vi "lfieldpanel_store_sequence.vi"(6 "dset_name":string, 7 "image_data":T1, 8 "error in (no error)":errorcluster, 9 "notes":string, 10 "Path":path, 11 "lightfield_panel in":refnum<class "lightfield_panel.lvclass">) -> (0 "error out":errorcluster, 3 "lightfield_panel out":refnum<class "lightfield_panel.lvclass">)   [LabVIEW 2015, in "lightfield_panel.lvclass"]
uses:
  lightfield_panel.lvclass
  lightfield_panel.lvclass/lightfield_panel.ctl
  lightfield_hdf5_logger_class/lfield_logger.lvclass
  lightfield_hdf5_logger_class/metadata_tdef.ctl
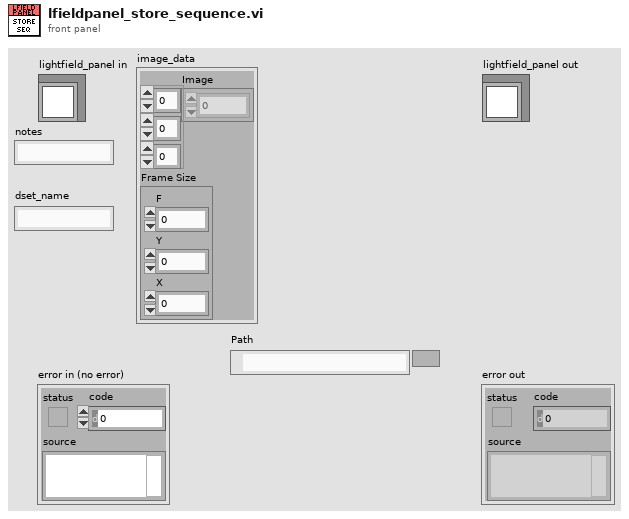
[diagram p1: front panel]
types:
  T1 = cluster{"Image":dbl[][][], "Frame Size":cluster{"F":i32, "Y":i32, "X":i32}}
  T2 = typedef "metadata_tdef.ctl" = cluster{"notes":string}
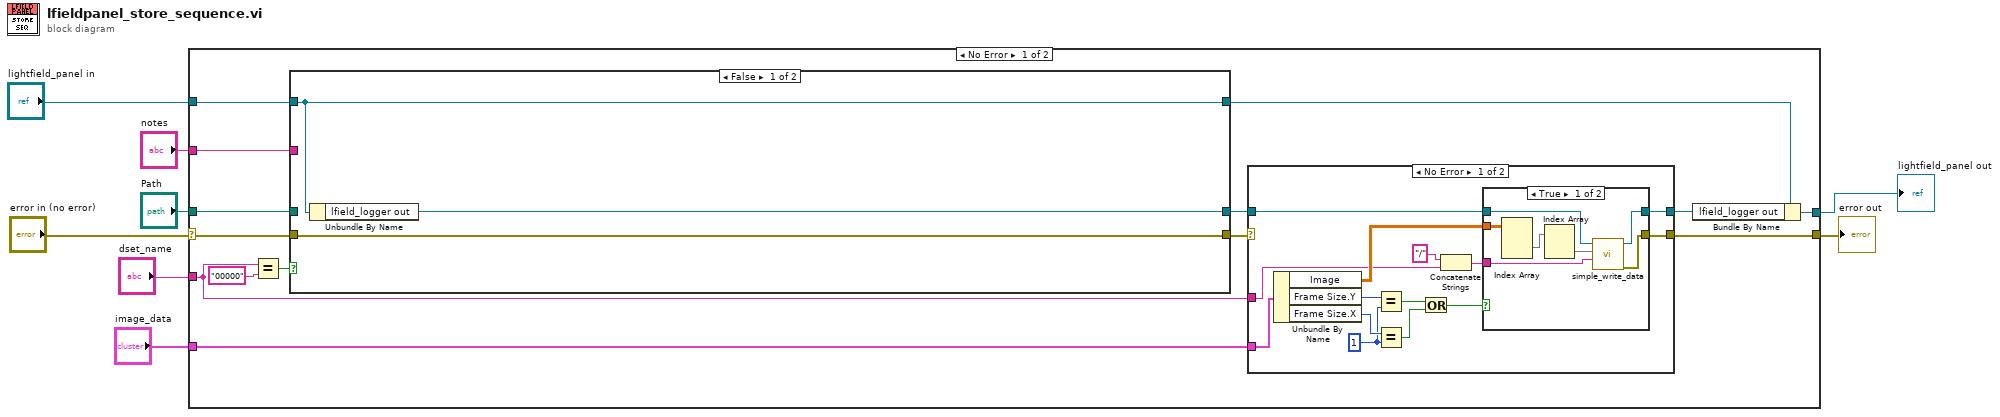
[diagram p0: block diagram]
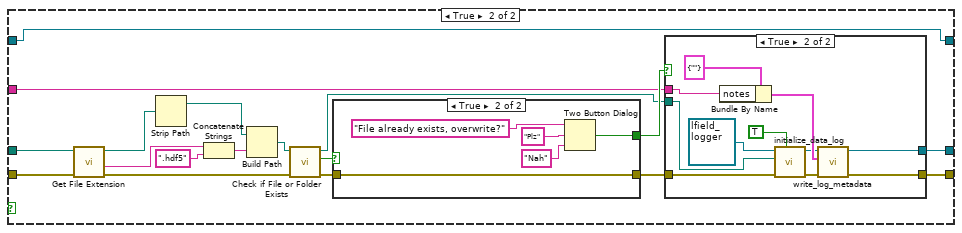
[diagram p2: hidden frame]
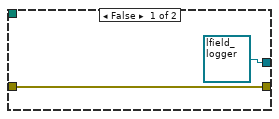
[diagram p3: hidden frame]
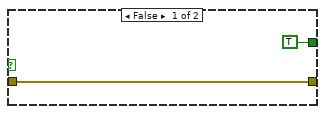
[diagram p4: hidden frame]
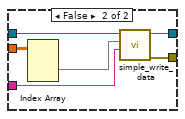
[diagram p5: hidden frame]
diagram:
  n1 = case shown="No Error" "error in (no error)" {
    selector: "error in (no error)" -> [w20 w94]
    tunnel: [w19 w94] -> w7
    tunnel: [w9 w93] -> w5
    tunnel: "lightfield_panel in" -> [w14 w93]
    tunnel: "image_data" -> [w22 _]
    tunnel: "Path" -> [w21 _]
    tunnel: "notes" -> [w12 _]
    tunnel: "dset_name" -> [w13 _]
    frame No Error {
      n2 = Equal?(x=w13, y="00000") -> (x = y?=w17:bool)
      n3 = case shown="False" w17 {
        tunnel: w21 -> [_ w43]
        tunnel: w20 -> [w25 w42]
        tunnel: [w25 w29] -> w16
        tunnel: [w24 w30] -> w15
        tunnel: w14 -> [w23 w27]
        tunnel: [w23 w27] -> w11
        tunnel: w12 -> [_ w26]
        frame False {
          n4 = Unbundle By Name(w23) -> ("lfield_logger out"=w24:refnum<class "lfield_logger.lvclass">)
        }
        frame True {
          n5 = call <vilib>:"Get File Extension.vi"("error in (no error)"=w42, "file"=w43) -> ("error out"=w35:errorcluster, "filename without extension"=w41:string, "dup file"=w39:path)  [unwired: 5 in, 2 out]
          n6 = Strip Path(path=w39) -> (stripped path=w38:path)  [unwired: 1 out]
          n7 = Concatenate Strings(w41, ".hdf5" ("string")) -> (w37:string)
          n8 = Build Path(base path=w38, name or relative path=w37) -> (appended path=w36:path)
          n9 = call <vilib>:"Check if File or Folder Exists.vi"("error in (no error)"=w35, "path"=w36) -> ("error out"=w33:errorcluster, "file or folder exists?"=w34:bool, "dup path"=w28:path)  [unwired: 7 in]
          n10 = case shown="True" w34 {
            tunnel: [TRUE ("T button?") w60] -> w32
            tunnel: w33 -> [w57 w59]
            tunnel: [w57 w59] -> w31
            frame False {
            }
            frame True {
              n11 = Two Button Dialog(message="File already exists, overwrite?", 1:"Nah" ("F button name (\"Cancel\")"), 2:"Plz" ("T button name (\"OK\")")) -> (T button?=w60:bool)
            }
          }
          n12 = case shown="True" w32 {
            tunnel: w31 -> [w44 w54]
            tunnel: [refnum<class "lfield_logger.lvclass"> refnum ("lfield_logger out") w48] -> w30
            tunnel: [w44 w47] -> w29
            tunnel: w28 -> [_ w53]
            tunnel: w26 -> [_ w46]
            frame False {
            }
            frame True {
              n13 = Bundle By Name(cluster=T2 {"notes"=""} ("output cluster"), "notes"=w46) -> (w51:T2)
              n14 = call-dynamic "initialize_data_log.vi"("Overwrite?"=TRUE, "error in (no error)"=w54, "Path"=w53, "lfield_logger in"=refnum<class "lfield_logger.lvclass"> refnum) -> ("error out"=w50:errorcluster, "lfield_logger out"=w49:refnum<class "lfield_logger.lvclass">)  [unwired: 6 in]
              n15 = call-dynamic "write_log_metadata.vi"("error in (no error)"=w50, "data"=w51, "lfield_logger in"=w49) -> ("error out"=w47:errorcluster, "lfield_logger out"=w48:refnum<class "lfield_logger.lvclass">)  [unwired: 7 in]
            }
          }
        }
      }
      n16 = case shown="No Error" w16 {
        selector: w16 -> [_ w91]
        tunnel: w22 -> [w77 _]
        tunnel: [w65 w91] -> w19
        tunnel: w15 -> [w69 w92]
        tunnel: w13 -> [w67 _]
        tunnel: [w64 w92] -> w10
        frame No Error {
          w74 = 1 ("y")
          n17 = Unbundle By Name(w77) -> ("Image"=w70:dbl[][][], "Frame Size.Y"=w76:i32, "Frame Size.X"=w75:i32)
          n18 = Equal?(x=w76, y=w74) -> (x = y?=w72:bool)
          n19 = Equal?(x=w75, y=w74) -> (x = y?=w73:bool)
          n20 = Or(x=w72, y=w73) -> (x .or. y?=w71:bool)
          n21 = Concatenate Strings("/" ("string"), w67) -> (w66:string)
          n22 = case shown="True" w71 {
            tunnel: w70 -> [w84 w90]
            tunnel: w66 -> [w81 w89]
            tunnel: [w80 w88] -> w64
            tunnel: [w79 w87] -> w65
            tunnel: w69 -> [w78 w85]
            frame True {
              n23 = Index Array(array=w84) -> (element=w83:dbl[][])  [unwired: 3 in]
              n24 = Index Array(array=w83) -> (element=w82:dbl[])  [unwired: 2 in]
              n25 = call "simple_write_data.vi"("path"=w81, "Data"=w82, "lfield_logger in"=w78) -> ("error out"=w79:errorcluster, "lfield_logger out"=w80:refnum<class "lfield_logger.lvclass">)  [unwired: 7 in]
            }
            frame False {
              n26 = Index Array(array=w90) -> (element=w86:dbl[][])  [unwired: 3 in]
              n27 = call "simple_write_data.vi"("path"=w89, "Data"=w86, "lfield_logger in"=w85) -> ("error out"=w87:errorcluster, "lfield_logger out"=w88:refnum<class "lfield_logger.lvclass">)  [unwired: 7 in]
            }
          }
        }
        frame Error {
        }
      }
      n28 = Bundle By Name(cluster=w11, "lfield_logger out"=w10) -> (w9:refnum<class "lightfield_panel.lvclass">)
    }
    frame Error {
    }
  }
  "error out" <- w7
  "lightfield_panel out" <- w5
